vi "Alias.vi"() -> ()   [LabVIEW 2024]
uses:
  <vilib>/Plug-In SDKs/Clients/Metadata/Alias.ctl
  <vilib>/Plug-In SDKs/Clients/Metadata/Alias Target Type.ctl
  <vilib>/Plug-In SDKs/Clients/Metadata/Operator.ctl
  <vilib>/Plug-In SDKs/Clients/Metadata/Extension.ctl
  <vilib>/Plug-In SDKs/Clients/Data Store V1/Data Store Client.lvlibp/API/Data Store V1/Test Result.ctl
  <vilib>/Plug-In SDKs/Clients/Metadata/Outcome.ctl
  <vilib>/Plug-In SDKs/Clients/Metadata Store V1/Metadata Store Client.lvlibp/API/Metadata Store V1/Create Operator.vi
  <vilib>/Plug-In SDKs/Clients/Metadata Store V1/Metadata Store Client.lvlibp/API/Metadata Store V1/Create Alias (Metadata - Operator).vi
  <vilib>/Plug-In SDKs/Clients/Metadata Store V1/Metadata Store Client.lvlibp/API/Metadata Store V1/Get Operator.vi
  <vilib>/Plug-In SDKs/Clients/Metadata/NI Metadata Types.lvlib
  <vilib>/Plug-In SDKs/Clients/Metadata Store V1/Metadata Store Client.lvlibp
  <vilib>/Plug-In SDKs/Clients/Data Store V1/Data Store Client.lvlibp
panel:
  out "query aliases results":T1[](array[typedef])
  out "get alias results":T1
  out "log":string
  out "error out":errorcluster
  # "Using Aliases\n\nThis example shows how to use the datastore API to...\n- Create aliases for metadata\n- Reference created aliases\n- Retrieve aliases\n- Delete aliases"
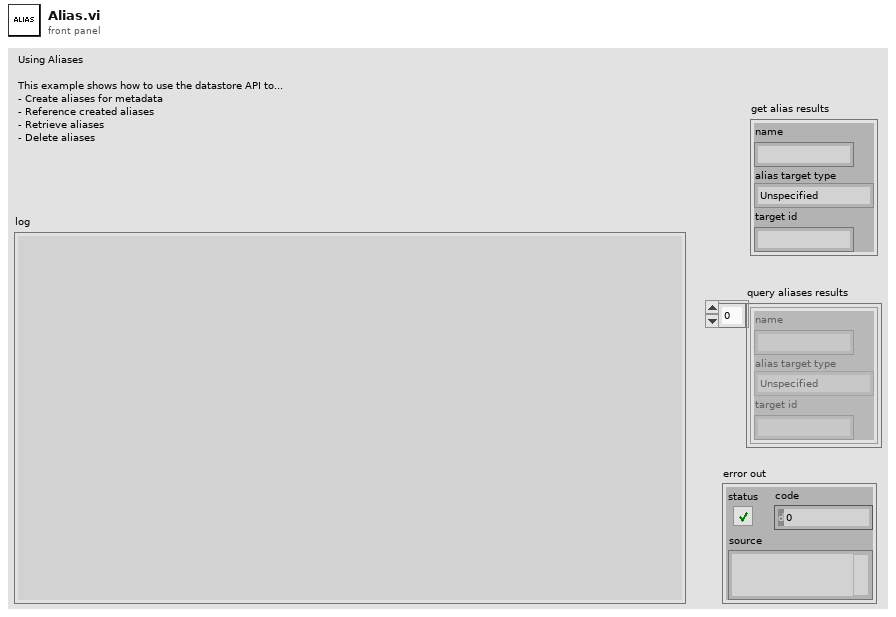
[diagram p1: front panel]
types:
  T1 = typedef "NI Metadata Types.lvlib/Alias.ctl" = cluster{"name":string, "alias target type":T2, "target id":string}
  T2 = typedef "NI Metadata Types.lvlib/Alias Target Type.ctl" = enum32{"Unspecified", "UUT Instance", "UUT", "Hardware Item", "Software Item", "Operator", "Test Description", "Test", "Test Station", "Test Adapter"}
  T3 = enum16{"Create Aliases", "Reference the Alias", "Retrieve Aliases", "Delete Aliases"}
  T4 = typedef "NI Metadata Types.lvlib/Operator.ctl" = cluster{"operator name":string, "role":string, "id":string, "link":string, "extensions":T5[], "schema id":string}
  T5 = typedef "NI Metadata Types.lvlib/Extension.ctl" = cluster{"name":string, "value":string}
  T6 = typedef "Data Store Client.lvlibp/Test Result.ctl" = cluster{"test result name":string, "start date time":timestamp, "end date time":timestamp, "outcome":T7, "test result id":string, "uut instance id":string, "operator id":string, "test station id":string, "test description id":string, "software item ids":string[], "hardware item ids":string[], "test adapter ids":string[], "link":string, "extensions":T5[], "schema id":string}
  T7 = typedef "NI Metadata Types.lvlib/Outcome.ctl" = enum32{"Unspecified", "Passed", "Failed", "Indeterminate"}
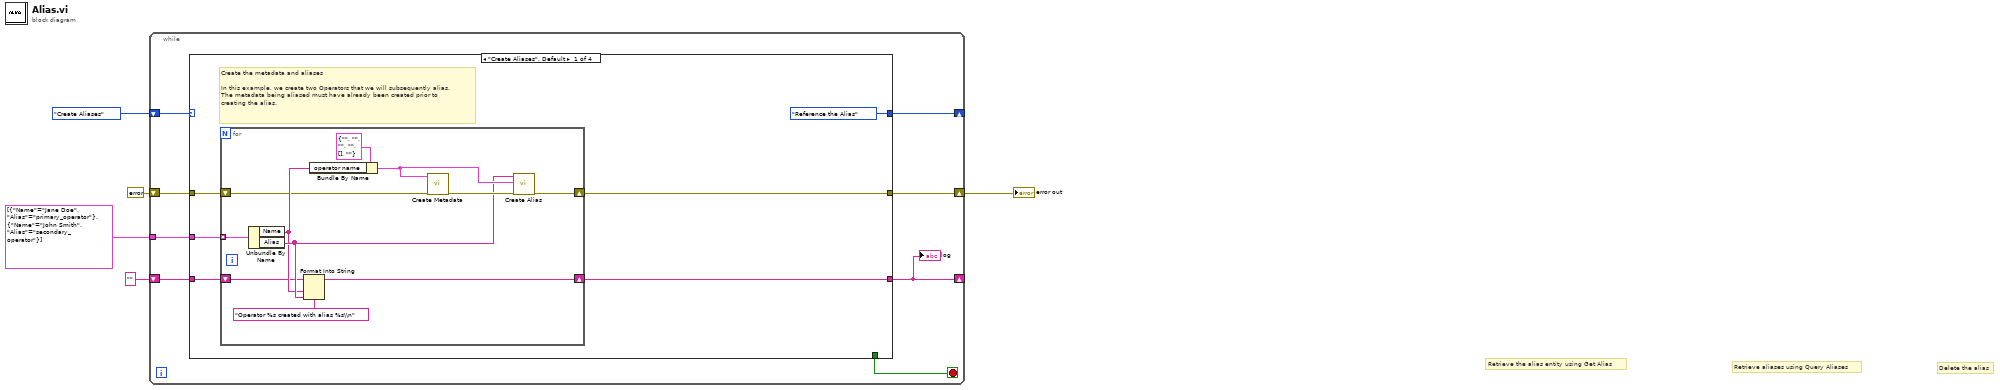
[diagram p0: block diagram]
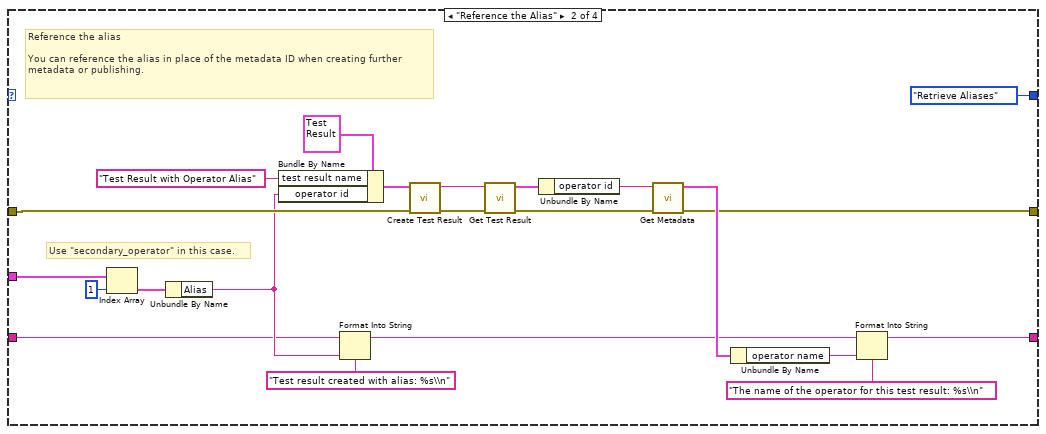
[diagram p2: hidden frame]
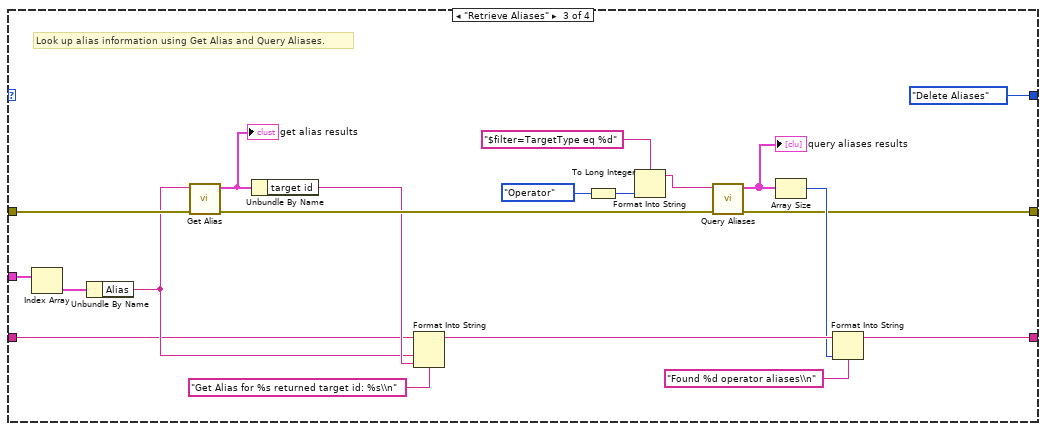
[diagram p3: hidden frame]
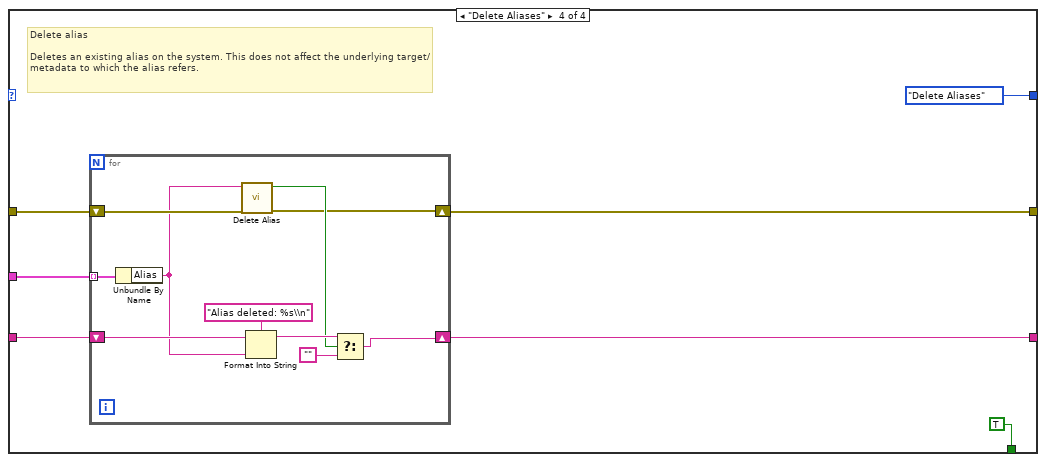
[diagram p4: hidden frame]
diagram:
  # "Delete the alias"
  # "Retrieve aliases using Query Aliases"
  # "Retrieve the alias entity using Get Alias"
  n1 = while {
    shift-right: [w7] -> _
    shift-left: T3."Create Aliases" -> [w13]
    shift-right: [w8] -> _
    shift-left: "" ("log") -> [w10]
    tunnel: cluster{"Name":string, "Alias":string}[] [{"Name"="Jane Doe", "Alias"="primary_operator"}, {"Name"="John Smith", "Alias"="secondary_operator"}] ("Array") -> [w12]
    shift-right: [w11] -> w2
    shift-left: errorcluster {"status"=FALSE, "code"=0, "source"=""} ("error out") -> [w9]
    stop <- w6 stop-if-true
    n2 = case shown="\"Create Aliases\", Default" w13 {
      tunnel: w12 -> [w19 w40 w59 w77]
      tunnel: [w18 w33 w54 w75] -> w11
      tunnel: w10 -> [w17 w36 w56 w79]
      tunnel: [w16 w32 w55 w76] -> w8
      tunnel: w9 -> [w15 w41 w60 w78]
      tunnel: [T3."Reference the Alias" T3."Retrieve Aliases" T3."Delete Aliases" T3."Delete Aliases"] -> w7
      tunnel: [_ _ _ TRUE] -> w6
      frame "Create Aliases", Default {
        # "Create the metadata and aliases\n\nIn this example, we create two Operators that we will subsequently alias. The metadata being aliased must have already been created prior to creating the alias."
        n3 = for {
          shift-right: [w30] -> w18
          shift-left: w15 -> [w20]
          tunnel: w19 -> [w26] mode=indexing
          shift-right: [w21] -> w16
          shift-left: w17 -> [w22]
          n4 = Unbundle By Name(w26) -> ("Name"=w23:string, "Alias"=w24:string)
          n5 = Format Into String(format string="Operator %s created with alias %s\\n", initial string=w22, w23, w24) -> (resulting string=w21:string)  [unwired: 1 in, 1 out]
          n6 = Bundle By Name(cluster=T4 {"operator name"="", "role"="", "id"="", "link"="", "extensions"=[], "schema id"=""} ("operator metadata"), "operator name"=w23) -> (w28:T4)
          n7 = call-poly <vilib>:"Create Metadata.vi"("error in"=w20, "operator metadata"=w28) -> ("error out"=w29:errorcluster)  [unwired: 8 in, 1 out]
          n8 = call-poly <vilib>:"Create Alias.vi"("error in"=w29, "operator"=w28, "alias name"=w24) -> ("error out"=w30:errorcluster)  [unwired: 7 in, 1 out]
        }
      }
      frame "Reference the Alias" {
        # "Reference the alias\n\nYou can reference the alias in place of the metadata ID when creating further metadata or publishing."
        # "Use \"secondary_operator\" in this case."
        n9 = Index Array(array=w40, index=1) -> (element=w38:cluster{"Name":string, "Alias":string})
        n10 = Unbundle By Name(w38) -> ("Alias"=w37:string)
        n11 = Bundle By Name(cluster=T6 {"test result name"="", "start date time"=timestamp(0 s since 1904-01-01), "end date time"=timestamp(0 s since 1904-01-01), "outcome"=enum."Unspecified", "test result id"="", "uut instance id"="", "operator id"="", "test station id"="", "test description id"="", "software item ids"=[], "hardware item ids"=[], "test adapter ids"=[], "link"="", "extensions"=[], "schema id"=""} ("test result"), "test result name"="Test Result with Operator Alias", "operator id"=w37) -> (w48:T6)
        n12 = Format Into String(format string="Test result created with alias: %s\\n", initial string=w36, w37) -> (resulting string=w34:string)  [unwired: 1 in, 1 out]
        n13 = call <vilib>:"Create Test Result.vi"("error in"=w41, "test result"=w48) -> ("error out"=w35:errorcluster, "test result id"=w52:string)  [unwired: 8 in]
        n14 = call <vilib>:"Get Test Result.vi"("error in"=w35, "test result id"=w52) -> ("error out"=w45:errorcluster, "test result"=w44:T6)  [unwired: 8 in]
        n15 = Unbundle By Name(w44) -> ("operator id"=w43:string)
        n16 = call-poly <vilib>:"Get Metadata.vi"("error in"=w45, "operator id"=w43) -> ("error out"=w33:errorcluster, "operator metadata"=w42:T4)  [unwired: 8 in]
        n17 = Unbundle By Name(w42) -> ("operator name"=w47:string)
        n18 = Format Into String(format string="The name of the operator for this test result: %s\\n", initial string=w34, w47) -> (resulting string=w32:string)  [unwired: 1 in, 1 out]
      }
      frame "Retrieve Aliases" {
        # "Look up alias information using Get Alias and Query Aliases."
        n19 = Index Array(array=w59) -> (element=w58:cluster{"Name":string, "Alias":string})  [unwired: 1 in]
        n20 = Unbundle By Name(w58) -> ("Alias"=w57:string)
        n21 = call <vilib>:"Get Alias.vi"("error in"=w60, "alias name"=w57) -> ("error out"=w65:errorcluster, "alias"=w61:T1)  [unwired: 8 in]
        "get alias results" <- w61
        n22 = Unbundle By Name(w61) -> ("target id"=w63:string)
        n23 = Format Into String(format string="Get Alias for %s returned target id: %s\\n" ("odata query"), initial string=w56, w57, w63) -> (resulting string=w72:string)  [unwired: 1 in, 1 out]
        n24 = To Long Integer(number=Alias_Target_Type."Operator" ("alias target type")) -> (32bit integer=w70:i32)
        n25 = Format Into String(format string="$filter=TargetType eq %d" ("odata query"), w70) -> (resulting string=w71:string)  [unwired: 2 in, 1 out]
        n26 = call <vilib>:"Query Aliases.vi"("error in"=w65, "odata query"=w71) -> ("error out"=w54:errorcluster, "aliases"=w66:T1[])  [unwired: 8 in]
        "query aliases results" <- w66
        n27 = Array Size(array=w66) -> (size(s)=w67:i32)
        n28 = Format Into String(format string="Found %d operator aliases\\n" ("odata query"), initial string=w72, w67) -> (resulting string=w55:string)  [unwired: 1 in, 1 out]
      }
      frame "Delete Aliases" {
        # "Delete alias\n\nDeletes an existing alias on the system. This does not affect the underlying target/metadata to which the alias refers."
        n29 = for {
          shift-right: [w83] -> w75
          shift-left: w78 -> [w84]
          tunnel: w77 -> [w82] mode=indexing
          shift-right: [w80] -> w76
          shift-left: w79 -> [w85]
          n30 = Unbundle By Name(w82) -> ("Alias"=w81:string)
          n31 = call <vilib>:"Delete Alias.vi"("error in"=w84, "alias name"=w81) -> ("error out"=w83:errorcluster, "deleted"=w88:bool)  [unwired: 8 in]
          n32 = Format Into String(format string="Alias deleted: %s\\n", initial string=w85, w81) -> (resulting string=w89:string)  [unwired: 1 in, 1 out]
          n33 = Select(t=w89, s=w88, f="") -> (s? t:f=w80:string)
        }
      }
    }
    "log" <- w8
  }
  "error out" <- w2
